vi "RM.getDeviceReservationDB.vi"(8 "error in":errorcluster, 10 "device name":string="deviceName", 11 "Item Ref in":T1 format="%.0x") -> (0 "error out":errorcluster, 1 "found":bool, 2 "reservation DB out":variant, 3 "Item Ref out":T1 format="%.0x")   [LabVIEW 2016, in "FPGA Addon Shared.lvlib"]
uses:
  FPGA Addon Shared.lvlib
  <vilib>/NI Veristand/Custom Device API/Custom Device Item Ref.ctl
  <vilib>/NI Veristand/Custom Device API/Get Item Property (Variant).vi
  <vilib>/NI VeriStand/Custom Device API/Custom Device API.lvlib
  <vilib>/NI VeriStand/Custom Device Tools/Custom Device Utility Library/Custom Device Utility Library.lvlib
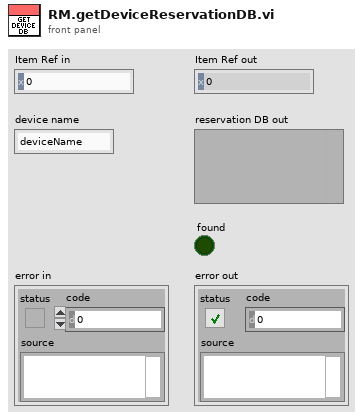
[diagram p1: front panel]
types:
  T1 = typedef "Custom Device API.lvlib/Custom Device Item Ref.ctl" = u64
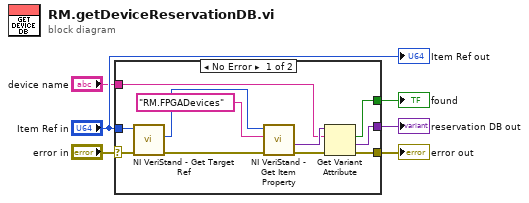
[diagram p0: block diagram]
diagram:
  n1 = case shown="No Error" "error in" {
    selector: "error in" -> [w11 w18]
    tunnel: "Item Ref in" -> [w17 _]
    tunnel: [w13 _] -> w6
    tunnel: [w12 _] -> w5
    tunnel: [w8 w18] -> w3
    tunnel: "device name" -> [w7 _]
    frame No Error {
      n2 = call <vilib>:"NI VeriStand - Get Target Ref.vi"("error in"=w11, "Item Ref in"=w17) -> ("error out"=w10:errorcluster, "Target Ref"=w16:T1)  [unwired: 6 in, 2 out]
      n3 = call-poly <vilib>:"NI VeriStand - Get Item Property.vi"("error in (no error)"=w10, "Property Name"="RM.FPGADevices", "Item Ref in"=w16) -> ("error out"=w9:errorcluster, "Value"=w14:variant)  [unwired: 5 in, 2 out]
      n4 = Get Variant Attribute(Variant=w14, name=w7, error in=w9) -> (found=w12:bool, value=w13:variant, error out=w8:errorcluster)  [unwired: 1 in, 1 out]
    }
    frame Error {
    }
  }
  "reservation DB out" <- w6
  "found" <- w5
  "error out" <- w3
  "Item Ref out" <- "Item Ref in"
